vi "2 ch.vi"() -> ()   [LabVIEW 2015]
uses:
  <instrlib>/Keithley 27XX/Public/Data/Read Multiple Direct.vi
  <instrlib>/Keithley 27XX/Keithley 27XX.lvlib
panel:
  out "output array":dbl[](array[numeric])
  out "VISA resource name out 2":refnum<visa-resource-name>
  in  "Number of channels":i32
  in  "VISA resource name out":refnum<visa-resource-name>
  out "error out 2":errorcluster
  in  "error out":errorcluster
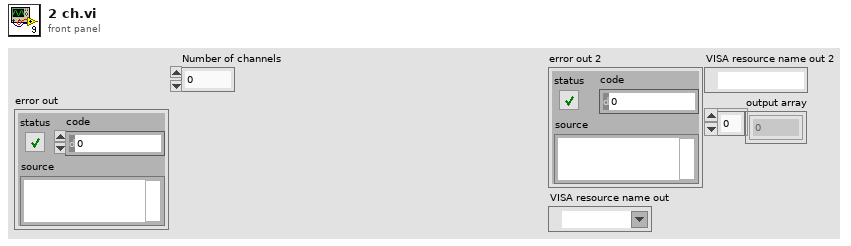
[diagram p1: front panel]
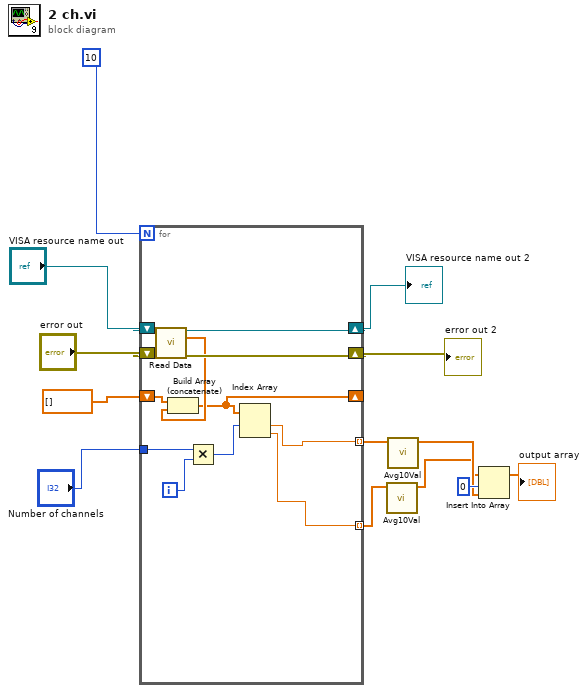
[diagram p0: block diagram]
diagram:
  n1 = for {
    N: 10 -> [_]
    shift-right: [w24] -> w12
    shift-left: "VISA resource name out" -> [w23]
    shift-right: [w25] -> w13
    shift-left: "error out" -> [w22]
    shift-right: [w16] -> _
    shift-left: dbl[] [] -> [w21]
    tunnel: "Number of channels" -> [w18]
    tunnel: [w15] -> w8 mode=indexing
    tunnel: [w14] -> w7 mode=indexing
    i -> [w19]
    n2 = call-poly <instrlib>:"Read Data.vi"("VISA resource name"=w23, "error in (no error)"=w22) -> ("VISA resource name out"=w24:refnum<visa-resource-name>, "Measurement Data"=w20:dbl[], "error out"=w25:errorcluster)  [unwired: 8 in, 3 out]
    n3 = Build Array (concatenate)(w21, w20) -> (w16:dbl[])
    n4 = Multiply(x=w18, y=w19) -> (x*y=w17:i32)
    n5 = Index Array(array=w16, index #1=w17) -> (element #1=w15:dbl, element #2=w14:dbl)  [unwired: 1 in]
  }
  "error out 2" <- w13
  "VISA resource name out 2" <- w12
  n6 = call "Avg10Val.vi"("element"=w7) -> ("Means of 10"=w5:dbl[])  [unwired: 10 in]
  n7 = call "Avg10Val.vi"("element"=w8) -> ("Means of 10"=w6:dbl[])  [unwired: 10 in]
  n8 = Insert Into Array(array=w5, index=0, new element=w6) -> (→"output array":dbl[])
